vi "FullAlign.vi"(0 "Joystick 0":dbl, 5 "Joystick 1":dbl, 7 "Distance":dbl, 9 "Angle":dbl, 11 "Button":bool=TRUE) -> (4 "Right Motor":dbl, 6 "Left Motor":dbl, 15 "output cluster":T1)   [LabVIEW 2016]
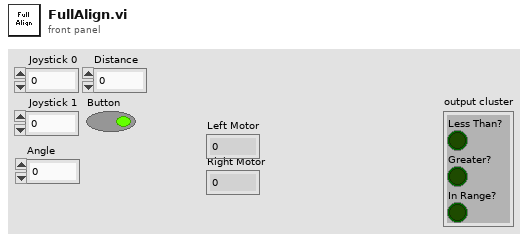
[diagram p1: front panel]
types:
  T1 = cluster{"Less Than? ":bool, "Greater?":bool, "In Range?":bool}
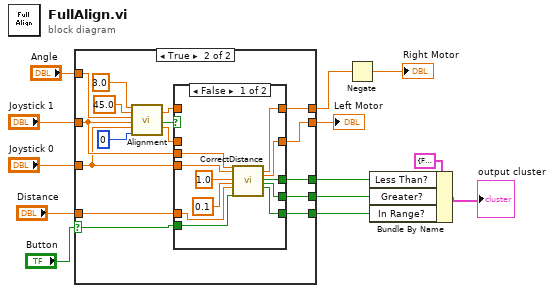
[diagram p0: block diagram]
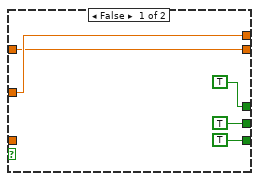
[diagram p2: hidden frame]
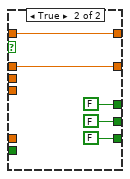
[diagram p3: hidden frame]
diagram:
  n1 = case shown="True" "Button" {
    selector: "Button" -> [_ w24]
    tunnel: "Joystick 1" -> [w17 w29]
    tunnel: "Joystick 0" -> [w18 w28]
    tunnel: [w17 w34] -> w6
    tunnel: [w18 w33] -> w8
    tunnel: "Angle" -> [_ w31]
    tunnel: [TRUE w23] -> w3
    tunnel: [TRUE w22] -> w4
    tunnel: [TRUE w21] -> w2
    tunnel: "Distance" -> [_ w20]
    frame False {
    }
    frame True {
      n2 = call "Alignment.vi"("Range"=3.0, "Target"=45.0, "Gyroscope Angle"=w31, "RightMotorSpeed"=w29, "LeftMotorSpeed"=w28, "POV"=0) -> ("Right Motor"=w27:dbl, "LeftAndRight?"=w25:bool, "Left Motor"=w26:dbl)  [unwired: 11 in]
      n3 = case shown="False" w25 {
        tunnel: w29 -> [w41 _]
        tunnel: w28 -> [w42 _]
        tunnel: [w40 w49] -> w34
        tunnel: [w39 w50] -> w33
        tunnel: w24 -> [w43 _]
        tunnel: w27 -> [_ w50]
        tunnel: w26 -> [_ w49]
        tunnel: [w38 FALSE] -> w23
        tunnel: [w37 FALSE] -> w22
        tunnel: [w36 FALSE] -> w21
        tunnel: w20 -> [w35 _]
        frame False {
          n4 = call "CorrectDistance.vi"("JoyStick 1"=w41, "JoyStick 2"=w42, "CenterPoint"=1.0, "Range"=0.1, "Distance"=w35, "Button"=w43) -> ("Right Motor"=w39:dbl, "Left Motor"=w40:dbl, "Less than"=w37:bool, "Greater"=w38:bool, "In Range?"=w36:bool)  [unwired: 16 in, 1 out]
        }
        frame True {
        }
      }
    }
  }
  "Left Motor" <- w6
  n5 = Negate(x=w8) -> (-x=→"Right Motor":dbl)
  n6 = Bundle By Name(cluster=T1 {"Less Than? "=FALSE, "Greater?"=FALSE, "In Range?"=FALSE} ("input cluster"), "Less Than?"=w4, "Greater?"=w3, "In Range?"=w2) -> (→"output cluster":T1)
